vi "New Count.vi"(10 "New Count":i32, 11 "API in":refnum<class "Data Generator API.lvclass">) -> ()   [LabVIEW 2024, in "Data Generator API.lvclass"]
uses:
  Data Generator API/Data Generator API.lvclass
  C:/Users/320141162/Desktop/DUTLug3/API/API.lvclass
  Message.ctl
  API.lvclass/API.ctl
  API.lvclass
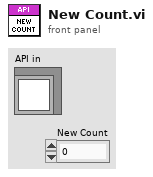
[diagram p1: front panel]
types:
  T1 = typedef "API.lvclass/Message.ctl" = cluster{"Name":string, "Data":variant}
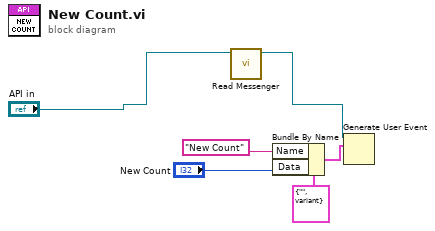
[diagram p0: block diagram]
diagram:
  n1 = call "Read Messenger.vi"("API in"="API in") -> ("Messenger"=w1:refnum<user-event>)  [unwired: 10 in]
  n2 = Bundle By Name(cluster=T1 {"Name"="", "Data"=variant} ("Message"), "Name"="New Count", "Data"="New Count") -> (w6:T1)
  n3 = Generate User Event(user event=w1, event data cluster=w6) -> ()  [unwired: 2 in, 2 out]
